vi "Pasco Bang Bang Control.vi"(9 "K":dbl, 10 "Current Power":dbl(slide) scale=-1.0..1.0, 11 "Setpoint":dbl(slide) scale=-1.0..1.0) -> (3 "power":dbl)   [LabVIEW 2012]
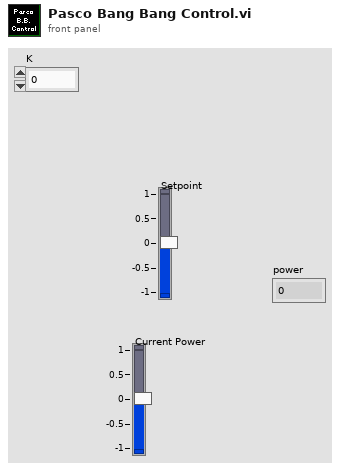
[diagram p1: front panel]
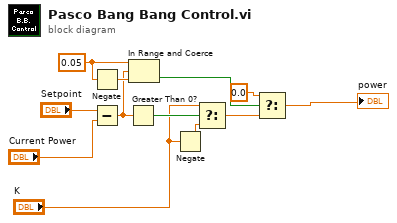
[diagram p0: block diagram]
diagram:
  w10 = 0.05 ("x")
  n1 = Negate(x=w10) -> (-x=w11:dbl)
  n2 = Subtract(x="Setpoint", y="Current Power") -> (x-y=w5:dbl)
  n3 = Greater Than 0?(x=w5) -> (x > 0?=w4:bool)
  n4 = In Range and Coerce(upper limit=w10, x=w5, lower limit=w11) -> (In Range?=w9:bool)  [unwired: 1 out]
  n5 = Negate(x="K") -> (-x=w2:dbl)
  n6 = Select(t="K", s=w4, f=w2) -> (s? t:f=w3:dbl)
  n7 = Select(t=0.0, s=w9, f=w3) -> (s? t:f=→"power":dbl)
